vi "GetSwerveAbsoluteAzimuth.vi"(0 "Relative Position (Raw Sensor Units)":i32) -> (1 "Azimuth Position (deg) [-180,+180]":dbl, 2 "Current Unwrapped Angle (deg) [-Inf,+Inf]":dbl)   [LabVIEW 2020]
doc: "Converts the relative azimuth encoder reading to an absolute azimuth angle."
uses:
  GlobalDrivebase.vi
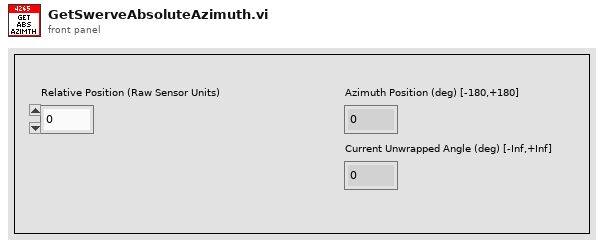
[diagram p1: front panel]
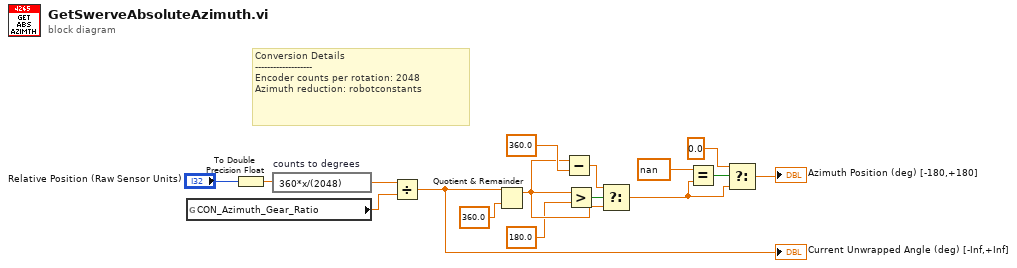
[diagram p0: block diagram]
diagram:
  # "Conversion Details\n-------------------\nEncoder counts per rotation: 2048\nAzimuth reduction: robotconstants"
  n1 = global read "GlobalDrivebase.vi" "CON_Azimuth_Gear_Ratio"() -> (w1:dbl)
  n2 = To Double Precision Float(number="Relative Position (Raw Sensor Units)") -> (double precision float=w15:dbl)
  n3 = expression code="360*x/(2048)" "counts to degrees"(w15) -> (w3:dbl)
  n4 = Divide(x=w3, y=w1) -> (x/y=w2:dbl)
  "Current Unwrapped Angle (deg) [-Inf,+Inf]" <- w2
  n5 = Quotient & Remainder(x=w2, y=360.0) -> (x-y*floor(x/y)=w12:dbl)  [unwired: 1 out]
  n6 = Subtract(x=w12, y=360.0) -> (x-y=w13:dbl)
  n7 = Greater?(x=w12, y=180.0) -> (0:w11:bool)
  n8 = Select(t=w13, s=w11, f=w12) -> (s? t:f=w6:dbl)
  n9 = Equal?(x=nan, y=w6) -> (x = y?=w7:bool)
  n10 = Select(t=0.0, s=w7, f=w6) -> (s? t:f=→"Azimuth Position (deg) [-180,+180]":dbl)
